vi "calc_moved direction.vi"(2 "rotate":cluster{"pitch":i32, "roll":i32, "yaw":i32}={"pitch"=-2, "roll"=-7, "yaw"=47} {"pitch" scale=-180.0..180.0; "roll" scale=-180.0..180.0; "yaw" scale=-180.0..180.0}, 3 "old pos":T1={"horizon"=1.1102230246251565e-15, "altitude"=-8.377522992154054, "distance"=4.440892098500626e-15} {"horizon" scale=-50.0..50.0; "altitude" scale=-100.0..200.0; "distance" scale=-200.0..200.0}) -> (0 "compass angle":dbl(slide)=46.75616374093017 scale=-180.0..180.0, 1 "new pos":T1={"horizon"=-0.7280075197732627, "altitude"=-8.41216235330034, "distance"=0.6846934831097519} {"horizon" scale=-50.0..50.0; "altitude" scale=-100.0..200.0; "distance" scale=-200.0..200.0})   [LabVIEW 2011]
uses:
  <vilib>/Analysis/baseanly.llb/Real A x B.vi
  <vilib>/Analysis/NI_AALBase.lvlib
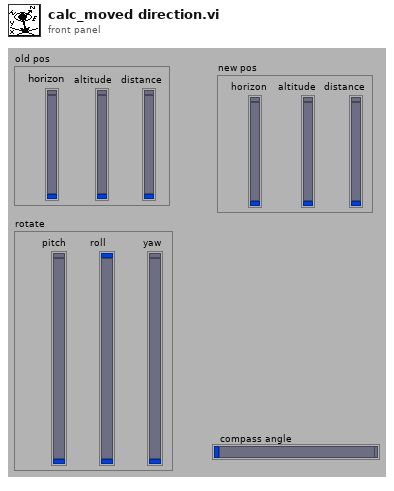
[diagram p1: front panel]
types:
  T1 = cluster{"horizon":dbl, "altitude":dbl, "distance":dbl}
  T2 = typedef "NI_Matrix.lvlib/RealMatrix.ctl" = dbl[][]
  T3 = cluster{"A x B[0]":dbl, "A x B[1]":dbl, "A x B[2]":dbl}
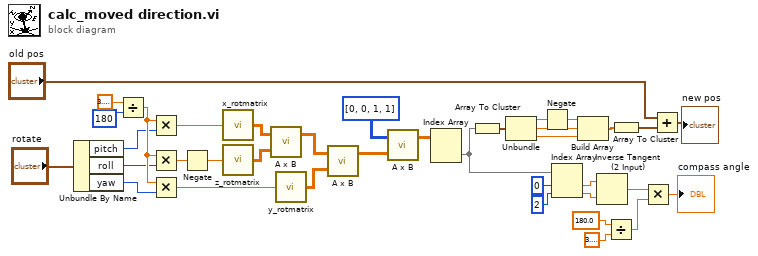
[diagram p0: block diagram]
diagram:
  n1 = Unbundle By Name("rotate") -> ("pitch"=w29:i32, "roll"=w28:i32, "yaw"=w27:i32)
  n2 = Divide(x=3.141592653589793, y=180) -> (x/y=w30:dbl)
  n3 = Multiply(x=w30, y=w29) -> (x*y=w10:dbl)
  n4 = Multiply(x=w30, y=w28) -> (x*y=w7:dbl)
  n5 = Multiply(x=w30, y=w27) -> (x*y=w3:dbl)
  n6 = Negate(x=w7) -> (-x=w6:dbl)
  n7 = call "x_rotmatrix.vi"("x-angle"=w10) -> ("x-matrix"=w9:dbl[][])
  n8 = call "z_rotmatrix.vi"("z-angle"=w6) -> ("z-matrix"=w8:dbl[][])
  n9 = call-poly <vilib>:"A x B.vi"("B"=w8, "A"=w9) -> ("A x B"=w5:T2)  [unwired: 1 out]
  n10 = call "y_rotmatrix.vi"("y-angle"=w3) -> ("y-matrix"=w4:dbl[][])
  n11 = call-poly <vilib>:"A x B.vi"("B"=w4, "A"=w5) -> ("A x B"=w2:T2)  [unwired: 1 out]
  n12 = call-poly <vilib>:"A x B.vi"("B"=w2, "A"=i32[][] [[0, 0, 1, 1]]) -> ("A x B"=w33:T2)  [unwired: 1 out]
  n13 = Index Array(array=w33) -> (element=w1:dbl[])  [unwired: 2 in]
  n14 = Array To Cluster(array=w1) -> (cluster=w34:T3)
  n15 = Unbundle(w34) -> ("A x B[0]"=w15:dbl, "A x B[1]"=w11:dbl, "A x B[2]"=w36:dbl)
  n16 = Negate(x=w15) -> (-x=w12:dbl)
  n17 = Index Array(array=w1, index #1=0 ("index"), index #2=2 ("index")) -> (element #1=w24:dbl, element #2=w23:dbl)
  n18 = Build Array(w12, w11, w36) -> (w35:dbl[])
  n19 = Inverse Tangent (2 Input)(1:w23, 2:w24) -> (0:w22:dbl)
  n20 = Divide(x=180.0 ("y"), y=3.141592653589793) -> (x/y=w19:dbl)
  n21 = Array To Cluster(array=w35) -> (cluster=w37:cluster{"[0]":dbl, "[1]":dbl, "[2]":dbl})
  n22 = Multiply(x=w22, y=w19) -> (x*y=→"compass angle":dbl)
  n23 = Add(x="old pos", y=w37) -> (x+y=→"new pos":cluster{dbl, dbl, dbl})
